vi "Calculate Derived Tractor Analog Variables.vi"(6 "Lower Tension Sub Data":dbl[](array[numeric]), 7 "Selected Tool":T1, 8 "Upper Tension Sub Data":dbl[](array[numeric])) -> (2 "Stroker Data Out":dbl[](array[numeric]))   [LabVIEW 2011]
uses:
  List of tools.ctl
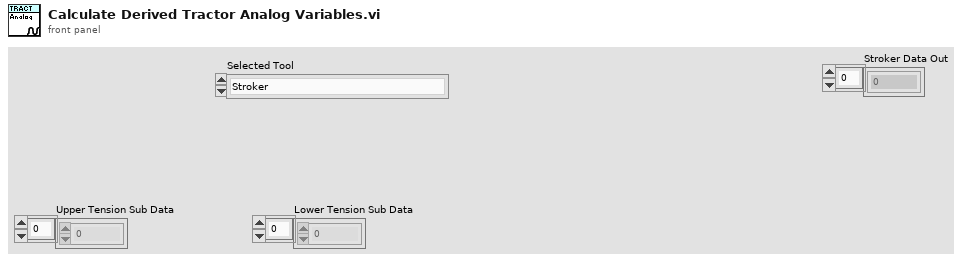
[diagram p1: front panel]
types:
  T1 = typedef "List of tools.ctl" = enum16{"Stroker", "Driller", "Tractor"}
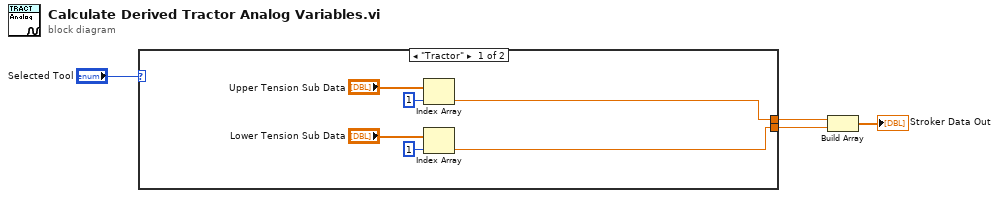
[diagram p0: block diagram]
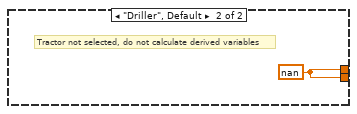
[diagram p2: hidden frame]
diagram:
  n1 = case shown="\"Tractor\"" "Selected Tool" {
    tunnel: [w6 w11] -> w2
    tunnel: [w5 w11] -> w1
    frame "Tractor" {
      n2 = Index Array(array="Upper Tension Sub Data", index=1) -> (element=w6:dbl)
      n3 = Index Array(array="Lower Tension Sub Data", index=1) -> (element=w5:dbl)
    }
    frame "Driller", Default {
      w11 = nan
      # "Tractor not selected, do not calculate derived variables"
    }
  }
  n4 = Build Array(w2, w1) -> (→"Stroker Data Out":dbl[])
